vi "263-264.vi"() -> ()   [LabVIEW 2020]
uses:
  C:/Program Files (x86)/National Instruments/LabVIEW 2020/examples/Connectivity/Python/support/PythonVersionsEnum.ctl
panel:
  out "字符串":string
  out "error out 2":cluster{"状态":bool, "代码":i32, "源":string} caption="错误输出"
  out "数值":i32
  out "非压缩地址 2":string
  out "压缩地址 2":string
  in  "error in (no error)":cluster{"状态":bool, "代码":i32, "源":string} caption="错误输入（无错误）"
  out "输出数组":string[](array[string])
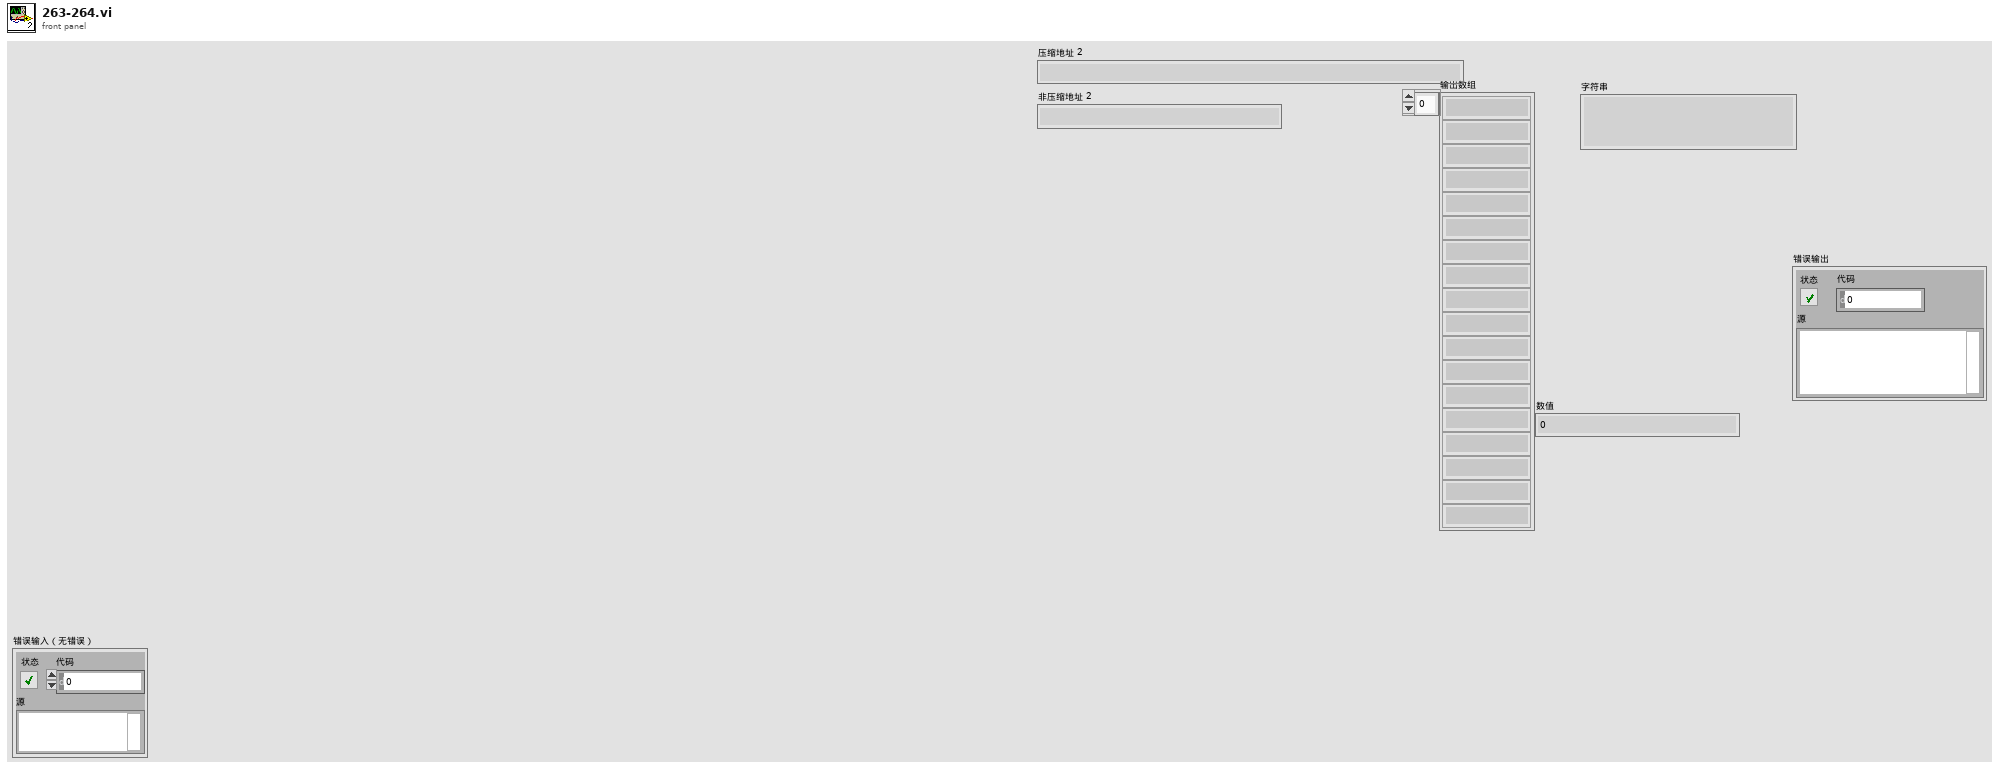
[diagram p1: front panel]
types:
  T1 = typedef "PythonVersionsEnum.ctl" = enum16{"2.7", "3.6"}
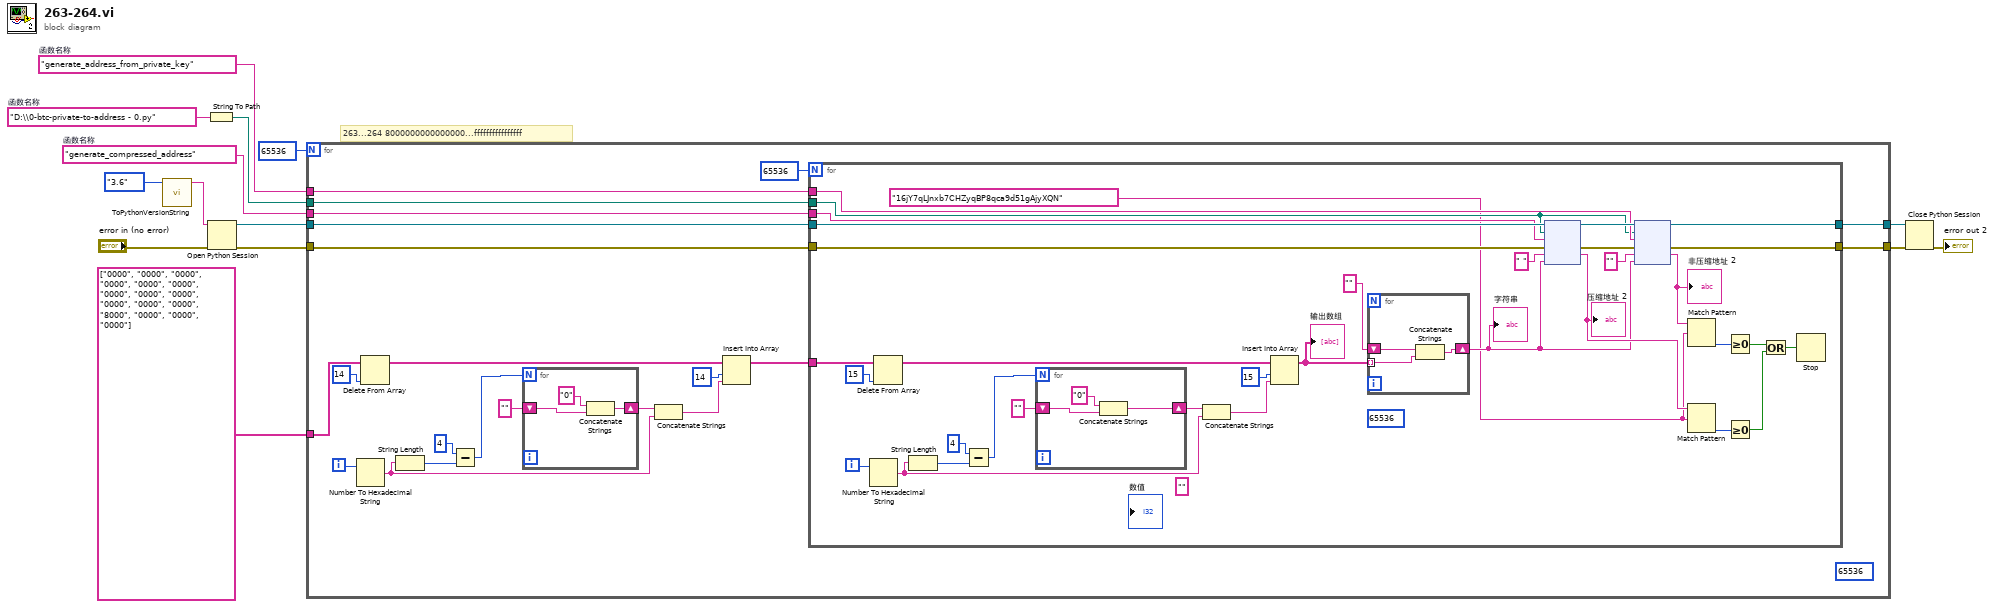
[diagram p0: block diagram]
diagram:
  w1 = "generate_compressed_address"  # 函数名称
  w3 = "D:\\0-btc-private-to-address - 0.py"  # 函数名称
  w4 = "generate_address_from_private_key"  # 函数名称
  # "263...264\t8000000000000000...ffffffffffffffff"
  n1 = call "ToPythonVersionString.vi"("Python版本"=PythonVersionsEnum."3.6") -> ("python版本字符串"=w12:string)  [unwired: 10 in]
  n2 = String To Path(string=w3) -> (path=w2:path)
  n3 = Open Python Session(python version=w12, 3:"error in (no error)") -> (session out=w9:refnum<k35>, error out=w8:errorcluster)  [unwired: 1 in]
  n4 = for {
    N: 65536 -> [_]
    tunnel: string[] ["0000", "0000", "0000", "0000", "0000", "0000", "0000", "0000", "0000", "0000", "0000", "0000", "8000", "0000", "0000", "0000"] ("数组") -> [w24]
    tunnel: w9 -> [w21]
    tunnel: w8 -> [w20]
    tunnel: [w19] -> w6
    tunnel: [w18] -> w5
    tunnel: w4 -> [w17]
    tunnel: w2 -> [w16]
    tunnel: w1 -> [w15]
    i -> [w26]
    (unwired) u32 65536 ("y")
    n5 = Number To Hexadecimal String(2:w26) -> (0:w27:string)  [unwired: 1 in]
    n6 = Delete From Array(array=w24, index=14 ("索引")) -> (array with subset deleted=w25:string[])  [unwired: 1 in, 1 out]
    n7 = String Length(string=w27) -> (length=w31:i32)
    n8 = Subtract(x=4 ("y"), y=w31) -> (x-y=w30:i32)
    n9 = for {
      N: w30 -> [_]
      shift-right: [w38] -> w28
      shift-left: "" -> [w37]
      n10 = Concatenate Strings("0" ("字符串"), w37) -> (w38:string)
    }
    n11 = Concatenate Strings(w28, w27) -> (w33:string)
    n12 = Insert Into Array(array=w25, index=14 ("索引"), new element=w33) -> (w23:string[])
    n13 = for {
      N: 65536 -> [_]
      tunnel: w23 -> [w66]
      tunnel: w21 -> [w56]
      tunnel: w20 -> [w55]
      tunnel: [w54] -> w19
      tunnel: [w53] -> w18
      tunnel: w17 -> [w42]
      tunnel: w16 -> [w41]
      tunnel: w15 -> [w40]
      i -> [w62]
      w39 = "16jY7qLJnxb7CHZyqBP8qca9d51gAjyXQN"
      (unwired) ""
      (unwired) u32 65536 ("y")
      n14 = Number To Hexadecimal String(2:w62) -> (0:w72:string)  [unwired: 1 in]
      n15 = Delete From Array(array=w66, index=15 ("索引")) -> (array with subset deleted=w64:string[])  [unwired: 1 in, 1 out]
      n16 = String Length(string=w72) -> (length=w68:i32)
      n17 = Subtract(x=4 ("y"), y=w68) -> (x-y=w69:i32)
      n18 = for {
        N: w69 -> [_]
        shift-right: [w78] -> w71
        shift-left: "" -> [w77]
        n19 = Concatenate Strings("0" ("字符串"), w77) -> (w78:string)
      }
      n20 = Concatenate Strings(w71, w72) -> (w63:string)
      n21 = Insert Into Array(array=w64, index=15 ("索引"), new element=w63) -> (w45:string[])
      "输出数组" <- w45
      n22 = for {
        tunnel: w45 -> [w75] mode=indexing
        shift-right: [w73] -> w43
        shift-left: "" -> [w74]
        n23 = Concatenate Strings(w74, w75) -> (w73:string)
      }
      "字符串" <- w43
      n24 = node(w56, w41, w40, w55, " ", w43) -> (w60:refnum<k35>, w59:errorcluster, w52:string)  [unwired: 1 in, 2 out]
      "压缩地址 2" <- w52
      n25 = node(w60, w41, w42, w59, "", w43) -> (w54:refnum<k35>, w53:errorcluster, w51:string)  [unwired: 1 in, 2 out]
      "非压缩地址 2" <- w51
      n26 = Match Pattern(string=w51, regular expression=w39) -> (offset past match=w50:i32)  [unwired: 1 in, 3 out]
      n27 = Match Pattern(string=w52, regular expression=w39) -> (offset past match=w49:i32)  [unwired: 1 in, 3 out]
      n28 = Greater Or Equal To 0?(x=w50) -> (x >= 0?=w48:bool)
      n29 = Greater Or Equal To 0?(x=w49) -> (x >= 0?=w47:bool)
      n30 = Or(x=w48, y=w47) -> (x .or. y?=w46:bool)
      n31 = Stop(stop? (T)=w46) -> ()
    }
  }
  n32 = Close Python Session(session in=w6, error in=w5) -> (11:→"error out 2":errorcluster)
